vi "myRIO_BRig_RT_TCP__quit.vi"(0 "input_hTCP":refnum<k5>, 3 "input_I_connected_TCP":bool, 11 "input_error":errorcluster) -> (4 "output_hTCP":refnum<k5>, 15 "output_error":errorcluster)   [LabVIEW 2014]
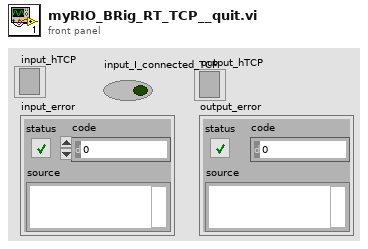
[diagram p1: front panel]
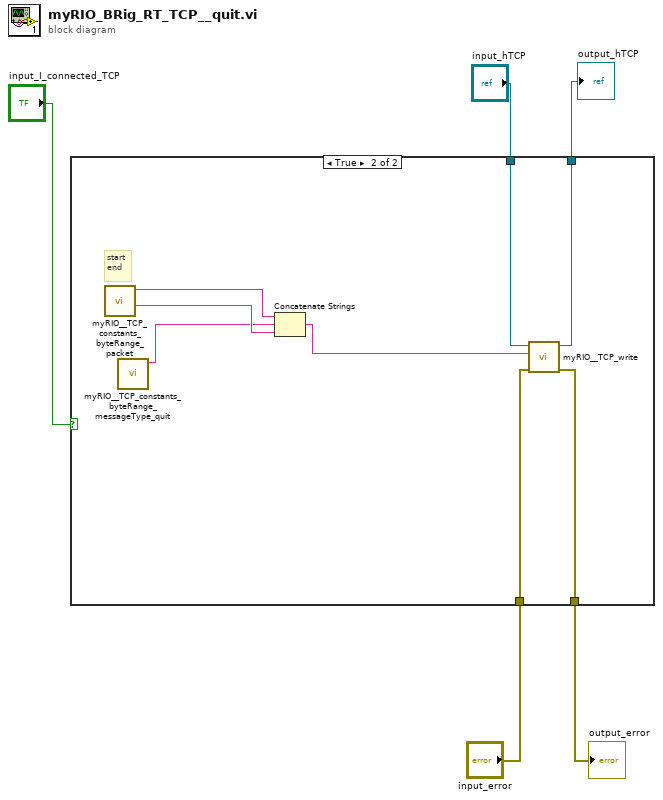
[diagram p0: block diagram]
diagram:
  n1 = case shown="True" "input_I_connected_TCP" {
    tunnel: "input_hTCP" -> [w7 w15]
    tunnel: "input_error" -> [w6 w14]
    tunnel: [w7 w13] -> w3
    tunnel: [w6 w12] -> w2
    frame False {
    }
    frame True {
      # "start\nend"
      n2 = call "myRIO__TCP_constants_byteRange_packet.vi"() -> ("output_end_char"=w10:string, "output_start_char"=w11:string)  [unwired: 8 in, 2 out]
      n3 = call "myRIO__TCP_constants_byteRange_messageType_quit.vi"() -> ("output_Quit_char"=w9:string)  [unwired: 10 in, 1 out]
      n4 = Concatenate Strings(w11, w9, w10) -> (w8:string)
      n5 = call "myRIO__TCP_write.vi"("input_error"=w14, "input_packet"=w8, "input_hTCP"=w15) -> ("output_error"=w12:errorcluster, "output_hTCP"=w13:refnum<k5>)  [unwired: 6 in, 1 out]
    }
  }
  "output_hTCP" <- w3
  "output_error" <- w2
